vi "Calculate State.vi"(9 "State":bool, 10 "Channel":T1, 11 "MCP23017 in":refnum<class "MCP23017.lvclass">) -> (3 "MCP23017 out":refnum<class "MCP23017.lvclass">)   [LabVIEW 2020, in "MCP23017.lvclass"]
uses:
  MCP23017.lvclass
  GPIO Channel.ctl
  MCP23017.lvclass/MCP23017.ctl
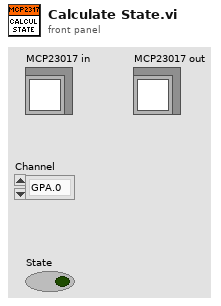
[diagram p1: front panel]
types:
  T1 = typedef "MCP23017.lvclass/GPIO Channel.ctl" = enum16{"GPA.0", "GPA.1", "GPA.2", "GPA.3", "GPA.4", "GPA.5", "GPA.6", "GPA.7", "GPB.0", "GPB.1", "GPB.2", "GPB.3", "GPB.4", "GPB.5", "GPB.6", "GPB.7"}
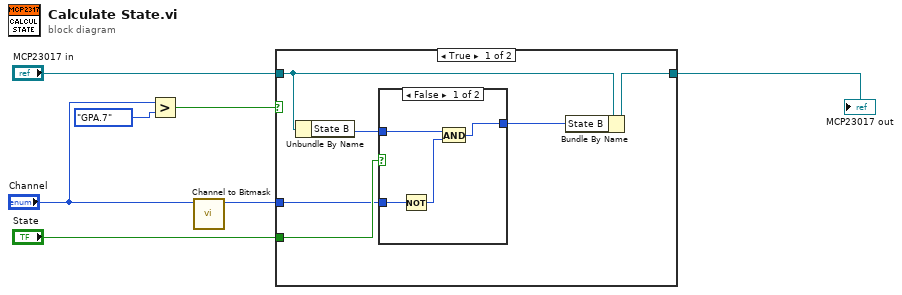
[diagram p0: block diagram]
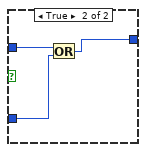
[diagram p2: hidden frame]
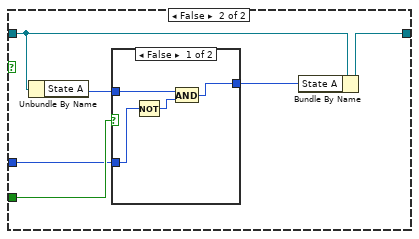
[diagram p3: hidden frame]
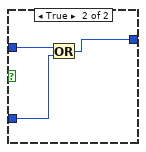
[diagram p4: hidden frame]
diagram:
  n1 = Greater?(x="Channel", y=GPIO_Channel."GPA.7" ("Channel")) -> (0:w1:bool)
  n2 = call "Channel to Bitmask.vi"("Channel"="Channel") -> ("Numeric"=w5:u8)  [unwired: 10 in]
  n3 = case shown="True" w1 {
    tunnel: "State" -> [w13 w26]
    tunnel: [w12 w25] -> w6
    tunnel: w5 -> [w10 w23]
    tunnel: "MCP23017 in" -> [w8 w21]
    frame True {
      n4 = Unbundle By Name(w8) -> ("State B"=w9:u8)
      n5 = case shown="False" w13 {
        tunnel: w9 -> [w17 w20]
        tunnel: w10 -> [w16 w19]
        tunnel: [w14 w18] -> w11
        frame False {
          n6 = Not(x=w16) -> (.not. x?=w15:u8)
          n7 = And(x=w17, y=w15) -> (x .and. y?=w14:u8)
        }
        frame True {
          n8 = Or(x=w20, y=w19) -> (x .or. y?=w18:u8)
        }
      }
      n9 = Bundle By Name(cluster=w8, "State B"=w11) -> (w12:refnum<class "MCP23017.lvclass">)
    }
    frame False {
      n10 = Unbundle By Name(w21) -> ("State A"=w22:u8)
      n11 = case shown="False" w26 {
        tunnel: w22 -> [w30 w33]
        tunnel: w23 -> [w29 w32]
        tunnel: [w27 w31] -> w24
        frame False {
          n12 = Not(x=w29) -> (.not. x?=w28:u8)
          n13 = And(x=w30, y=w28) -> (x .and. y?=w27:u8)
        }
        frame True {
          n14 = Or(x=w33, y=w32) -> (x .or. y?=w31:u8)
        }
      }
      n15 = Bundle By Name(cluster=w21, "State A"=w24) -> (w25:refnum<class "MCP23017.lvclass">)
    }
  }
  "MCP23017 out" <- w6
